vi "Get String Value For JSON.vi"(4 "No Control Index":bool, 6 "String Is Path":bool, 7 "VI Reference":refnum<vi>, 8 "error in (no error)":errorcluster, 9 "Control Index":i32, 10 "Default Value":variant, 11 "GObject in":refnum<vi>) -> (0 "error out":errorcluster, 3 "Text":string)   [LabVIEW 2017, in "Front Panel Publisher.lvlib" / "String.lvclass"]
uses:
  String.lvclass
  Control_class/Control.lvclass
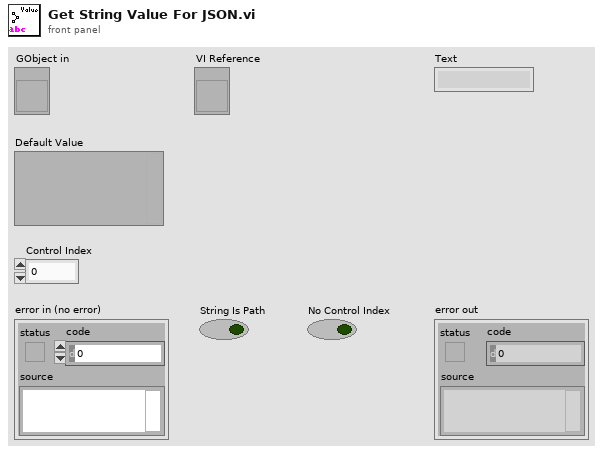
[diagram p1: front panel]
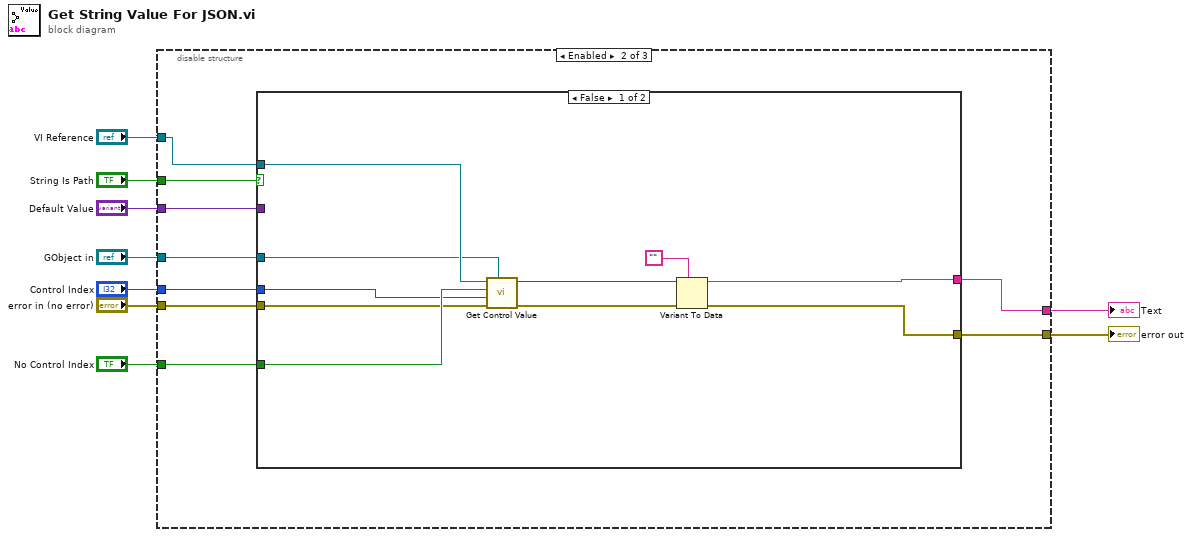
[diagram p0: block diagram]
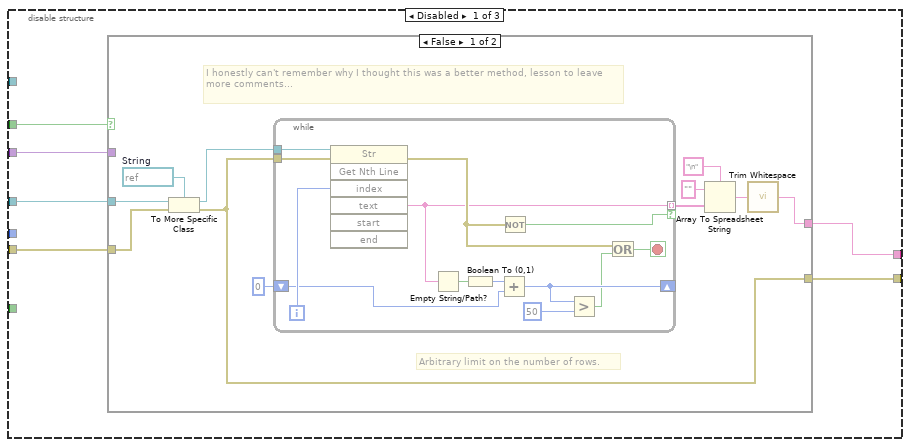
[diagram p2: hidden frame]
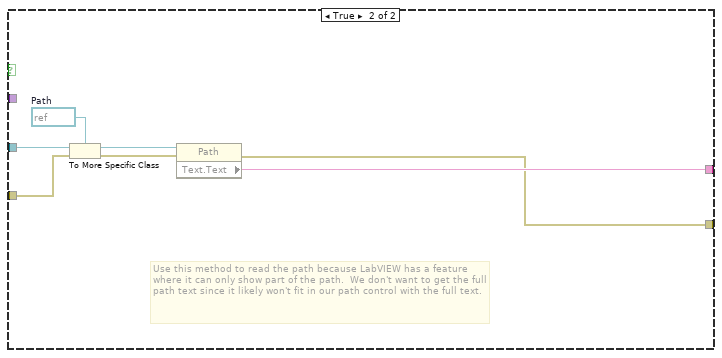
[diagram p3: hidden frame]
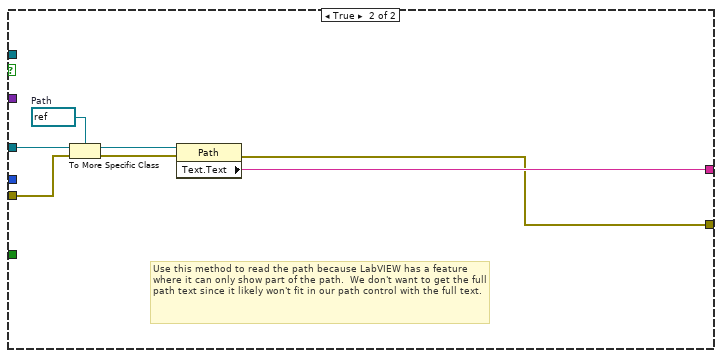
[diagram p4: hidden frame]
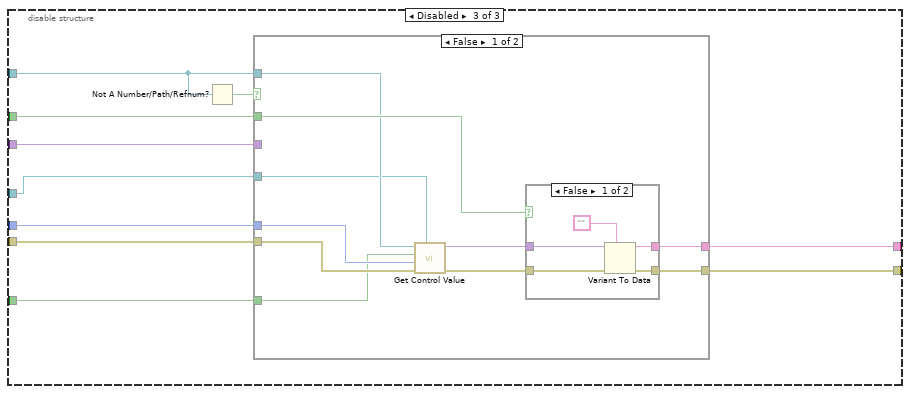
[diagram p5: hidden frame]
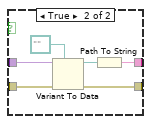
[diagram p6: hidden frame]
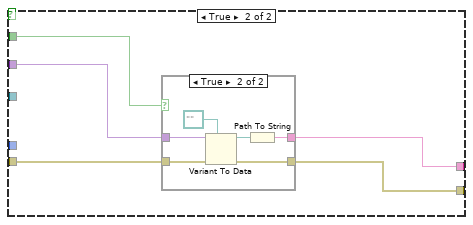
[diagram p7: hidden frame]
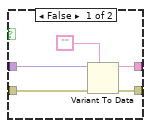
[diagram p8: hidden frame]
diagram:
  n1 = disable-structure shown="Enabled" {
    disable-tunnel: "GObject in" -> [w15 w55 w75]
    disable-tunnel: "String Is Path" -> [w14 w54 w82]
    disable-tunnel: [w13 w53 w81] -> w7
    disable-tunnel: "Default Value" -> [w12 w52 w77]
    disable-tunnel: "Control Index" -> [_ w47 w76]
    disable-tunnel: "VI Reference" -> [_ w49 w73]
    disable-tunnel: [w10 w50 w80] -> w2
    disable-tunnel: "error in (no error)" -> [w11 w51 w79]
    disable-tunnel: "No Control Index" -> [_ w48 w74]
    frame Disabled {
      n2 = case shown="False" w14 {
        tunnel: w12 -> [_ _]
        tunnel: [w20 w43] -> w13
        tunnel: w15 -> [w25 w46]
        tunnel: w11 -> [w17 w41]
        tunnel: [w16 w40] -> w10
        frame False {
          w26 = refnum<vi> refnum  # String
          # "I honestly can't remember why I thought this was a better method, lesson to leave more comments..."
          # "Arbitrary limit on the number of rows."
          n3 = To More Specific Class(target class=w26, reference=w25, error in=w17) -> (specific class reference=w21:refnum<vi>, error out=w16:errorcluster)
          n4 = while {
            tunnel: [w34] -> w24 mode=indexing if=w38
            tunnel: w21 -> [w37]
            tunnel: w16 -> [w36]
            shift-right: [w30] -> _
            shift-left: i16 0 -> [w31]
            i -> [w35]
            stop <- w28 stop-if-true
            n5 = invoke on="Invoke Node" class="Str" method="Get Nth Line"(reference=w37, error in=w36, "index"=w35) -> (error out=w39:errorcluster, "text"=w34:string)  [unwired: 4 in, 5 out]
            n6 = Empty String/Path?(string/path=w34) -> (empty?=w33:bool)
            n7 = Boolean To (0,1)(Boolean=w33) -> (0, 1=w32:i16)
            n8 = Add(x=w32, y=w31) -> (x+y=w30:i16)
            n9 = Not(x=w39) -> (.not. x?=w38:bool)
            n10 = Greater?(x=w30, y=i16 50) -> (0:w27:bool)
            n11 = Or(x=w39, y=w27) -> (x .or. y?=w28:bool)
          }
          n12 = Array To Spreadsheet String(delimiter (Tab)="\n", array=w24, 3:"" ("format string")) -> (spreadsheet string=w22:string)
          n13 = call <vilib>:"Trim Whitespace.vi"("string"=w22) -> ("trimmed string"=w20:string)  [unwired: 1 in]
        }
        frame True {
          w45 = refnum<vi> refnum  # Path
          # "Use this method to read the path because LabVIEW has a feature where it can only show part of the path.  We don't want to get the full path text since it likely won't fit in our path control with the full text."
          n14 = To More Specific Class(target class=w45, reference=w46, error in=w41) -> (specific class reference=w44:refnum<vi>, error out=w42:errorcluster)
          n15 = property class="Path"(reference=w44, error in=w42) -> (error out=w40:errorcluster, "Text.Text"=w43:string)  [unwired: 1 out]
        }
      }
    }
    frame Enabled {
      n16 = case shown="False" w54 {
        tunnel: w52 -> [_ _]
        tunnel: [w56 w69] -> w53
        tunnel: w55 -> [w61 w72]
        tunnel: w51 -> [w57 w67]
        tunnel: [w58 w66] -> w50
        tunnel: w49 -> [w62 _]
        tunnel: w48 -> [w60 _]
        tunnel: w47 -> [w59 _]
        frame False {
          n17 = call "Get Control Value.vi"("Control Reference"=w61, "error in (no error)"=w57, "Control Index"=w59, "No Control Index"=w60, "VI Reference"=w62) -> ("error out"=w63:errorcluster, "Variant"=w64:variant)  [unwired: 5 in]
          n18 = Variant To Data(error in=w63, type="", Variant=w64) -> (data=w56:string, error out=w58:errorcluster)
        }
        frame True {
          w71 = refnum<vi> refnum  # Path
          # "Use this method to read the path because LabVIEW has a feature where it can only show part of the path.  We don't want to get the full path text since it likely won't fit in our path control with the full text."
          n19 = To More Specific Class(target class=w71, reference=w72, error in=w67) -> (specific class reference=w70:refnum<vi>, error out=w68:errorcluster)
          n20 = property class="Path"(reference=w70, error in=w68) -> (error out=w66:errorcluster, "Text.Text"=w69:string)  [unwired: 1 out]
        }
      }
    }
    frame Disabled {
      n21 = Not A Number/Path/Refnum?(number/path/refnum=w73) -> (NaN/Path/Refnum?=w78:bool)
      n22 = case shown="False" w78 {
        tunnel: w76 -> [w89 _]
        tunnel: w82 -> [w92 w104]
        tunnel: [w91 w105] -> w81
        tunnel: [w90 w106] -> w80
        tunnel: w79 -> [w86 w108]
        tunnel: w73 -> [w88 _]
        tunnel: w77 -> [_ w107]
        tunnel: w75 -> [w87 _]
        tunnel: w74 -> [w83 _]
        frame False {
          n23 = call "Get Control Value.vi"("Control Reference"=w87, "error in (no error)"=w86, "Control Index"=w89, "No Control Index"=w83, "VI Reference"=w88) -> ("error out"=w85:errorcluster, "Variant"=w84:variant)  [unwired: 5 in]
          n24 = case shown="False" w92 {
            tunnel: w85 -> [w97 w103]
            tunnel: w84 -> [w96 w102]
            tunnel: [w94 w98] -> w91
            tunnel: [w93 w99] -> w90
            frame False {
              n25 = Variant To Data(error in=w97, type="", Variant=w96) -> (data=w94:string, error out=w93:errorcluster)
            }
            frame True {
              n26 = Variant To Data(error in=w103, type=path "", Variant=w102) -> (data=w100:path, error out=w99:errorcluster)
              n27 = Path To String(path=w100) -> (string=w98:string)
            }
          }
        }
        frame True {
          n28 = case shown="True" w104 {
            tunnel: w108 -> [w113 w119]
            tunnel: w107 -> [w112 w118]
            tunnel: [w110 w114] -> w105
            tunnel: [w109 w115] -> w106
            frame False {
              n29 = Variant To Data(error in=w113, type="", Variant=w112) -> (data=w110:string, error out=w109:errorcluster)
            }
            frame True {
              n30 = Variant To Data(error in=w119, type=path "", Variant=w118) -> (data=w116:path, error out=w115:errorcluster)
              n31 = Path To String(path=w116) -> (string=w114:string)
            }
          }
        }
      }
    }
  }
  "Text" <- w7
  "error out" <- w2
